vi "Control Loop Process.vi"(8 "error in (no error)":errorcluster, 9 "MainDirectionIn":string, 11 "Main Process Class in":refnum<class "MPC_AutoInspection.lvclass">) -> (0 "error out":errorcluster, 1 "MainDirectionOut":string, 2 "ProcessAction":string[](array[string]), 3 "Main Process Class out":refnum<class "MPC_AutoInspection.lvclass">)   [LabVIEW 2019, in "MPC_AutoInspection.lvclass"]
uses:
  MPC_AutoInspection.lvclass
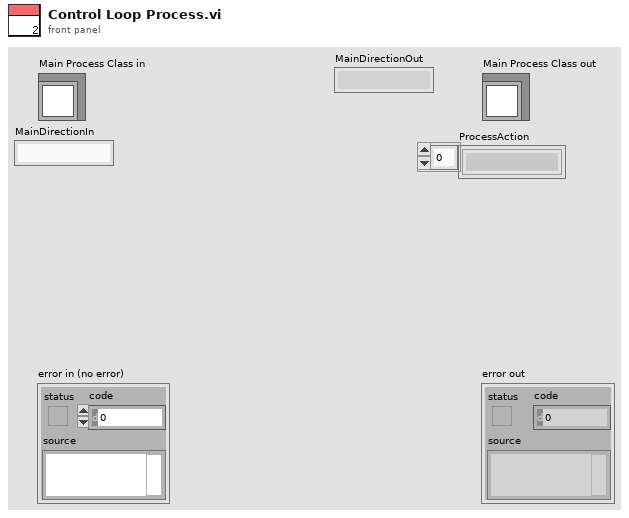
[diagram p1: front panel]
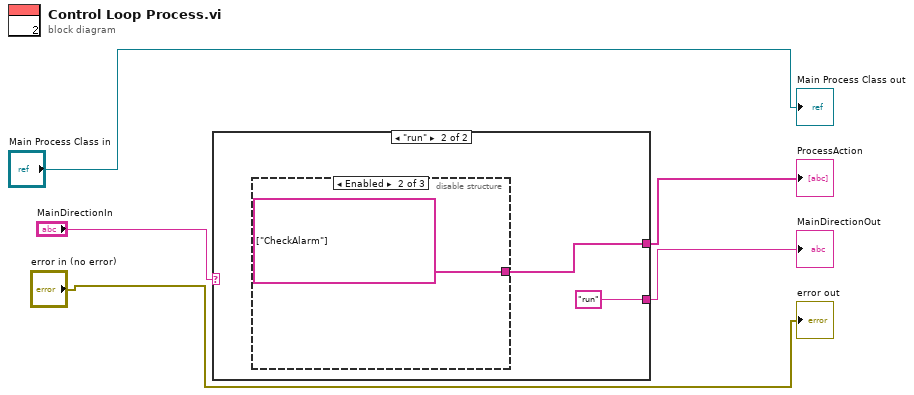
[diagram p0: block diagram]
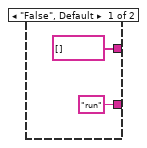
[diagram p2: hidden frame]
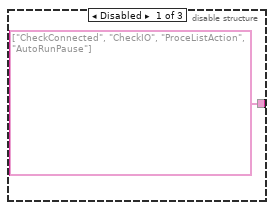
[diagram p3: hidden frame]
diagram:
  n1 = case shown="\"run\"" "MainDirectionIn" {
    tunnel: ["run" "run"] -> w4
    tunnel: [string[] [] w8] -> w3
    frame "False", Default {
    }
    frame "run" {
      n2 = disable-structure shown="Enabled" {
        disable-tunnel: [string[] ["CheckConnected", "CheckIO", "ProceListAction", "AutoRunPause"] string[] ["CheckAlarm"] _] -> w8
        frame Disabled {
        }
        frame Enabled {
        }
        frame Disabled {
        }
      }
    }
  }
  "MainDirectionOut" <- w4
  "ProcessAction" <- w3
  "error out" <- "error in (no error)"
  "Main Process Class out" <- "Main Process Class in"
